vi "UsrProfiles-Register user and profile in global.vi"(8 "error in":errorcluster, 9 "User Name":string, 11 "Profile name (no user prefix or file extension)":string) -> (0 "error out":errorcluster)   [LabVIEW 2017]
uses:
  Globals/gl_UsrProfiles globals.vi
  Global Variables/General Globals.vi
panel:
  out "Profile filename":string
  out "Profile filepath":path
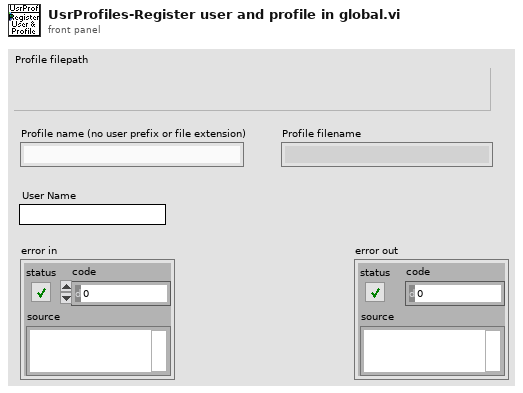
[diagram p1: front panel]
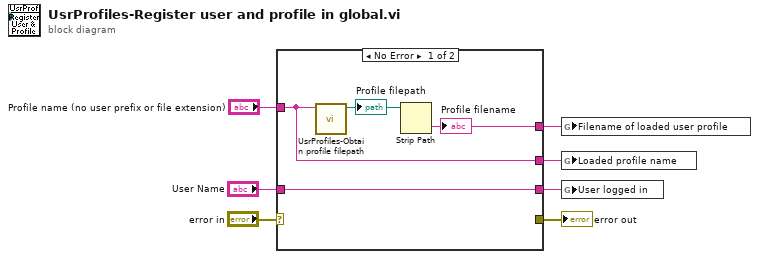
[diagram p0: block diagram]
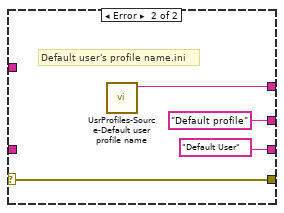
[diagram p2: hidden frame]
diagram:
  n1 = case shown="No Error" "error in" {
    selector: "error in" -> [_ w15]
    tunnel: [_ w15] -> w7
    tunnel: "Profile name (no user prefix or file extension)" -> [w8 _]
    tunnel: [w11 w12] -> w5
    tunnel: [w9 "Default User" ("User Name")] -> w2
    tunnel: "User Name" -> [w9 _]
    tunnel: [w8 "Default profile" ("Profile name (no user prefix or file extension)")] -> w1
    frame No Error {
      n2 = call "UsrProfiles-Obtain profile filepath.vi"("Profile name"=w8) -> ("Profile filepath"=w10:path)  [unwired: 9 in, 1 out]
      "Profile filepath" <- w10
      n3 = Strip Path(path=w10) -> (name=w11:string)  [unwired: 1 out]
      "Profile filename" <- w11
    }
    frame Error {
      # "Default user's profile name.ini"
      n4 = call "UsrProfiles-Source-Default user profile name.vi"() -> ("Default user's profile file name & extension"=w12:string)  [unwired: 11 in]
    }
  }
  "error out" <- w7
  n5 = global write "General Globals.vi" "Filename of loaded user profile"(w5) -> ()
  n6 = global write "gl_UsrProfiles globals.vi" "Loaded profile name"(w1) -> ()
  n7 = global write "gl_UsrProfiles globals.vi" "User logged in"(w2) -> ()
